vi "DSP_conditioning_Rx.bkp - Copy.vi"(4 "rx.output sample rate":fxp<+,48,1>=1.0, 5 "rx.input valid":bool, 6 "rx.frequency shift":fxp<+/-,48,0> format="%#.48g", 7 "rx.reset":bool, 8 "rx.phase":fxp<+/-,21,0>, 9 "rx.delay":fxp<+/-,16,0>, 10 "rx.impairments":T2={"inline gain I"=0.9999923706054688, "inline gain Q"=0.9999923706054688, "cross gain I"=0.0, "cross gain Q"=0.0, "pre-gain offset I"=0.0, "pre-gain offset Q"=0.0, "post-gain offset I"=0.0, "post-gain offset Q"=0.0}, 11 "IQ data":T1) -> (1 "rx.dsp reset done":bool, 2 "output valid":bool, 3 "data out":T1)   [LabVIEW 2017]
uses:
  <instrlib>/_niInstr/DSP/v1/Shared/Public/IQ Impairments.ctl
  <instrlib>/_niInstr/DSP/v1/Shared/Public/IQ Data.ctl
  <instrlib>/_niInstr/DSP/v1/FPGA/Public/Sub VIs/IQ Impairments/IQ Impairments - 1 spc.vi
  <instrlib>/_niInstr/DSP/v1/FPGA/Public/Sub VIs/Frequency Shift/Frequency Shift - 1 spc.vi
  <instrlib>/_niInstr/DSP/v1/FPGA/Public/Sub VIs/Data Conversion/IQ to U32 - 1 spc - S18.1.vi
  <instrlib>/_niInstr/DSP/v1/FPGA/niInstr DSP v1 FPGA.lvlib
  <instrlib>/_niInstr/Basic Elements/v1/FPGA/niInstr Basic Elements v1 FPGA.lvlib
  <instrlib>/_niInstr/DSP/v1/FPGA/Public/Sub VIs/Fractional Decimator/Fractional Decimator - 1 spc - 2x oc.vi
  <instrlib>/_niInstr/DSP/v1/Shared/niInstr DSP v1 Shared.lvlib
panel:
  out "U32 data":u32
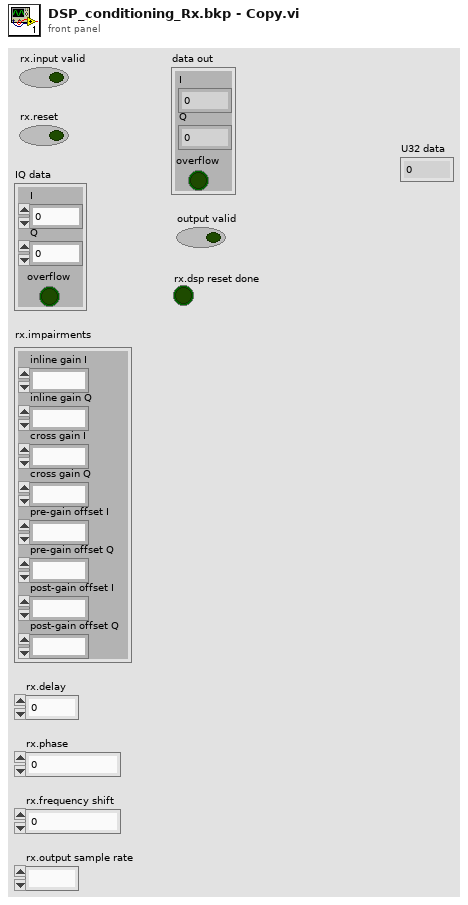
[diagram p1: front panel]
types:
  T1 = typedef "niInstr DSP v1 Shared.lvlib/IQ Data.ctl" = cluster{"I":fxp<+/-,18,1>, "Q":fxp<+/-,18,1>, "overflow":bool}
  T2 = typedef "niInstr DSP v1 Shared.lvlib/IQ Impairments.ctl" = cluster{"inline gain I":fxp<+/-,18,1>, "inline gain Q":fxp<+/-,18,1>, "cross gain I":fxp<+/-,18,1>, "cross gain Q":fxp<+/-,18,1>, "pre-gain offset I":fxp<+/-,18,1>, "pre-gain offset Q":fxp<+/-,18,1>, "post-gain offset I":fxp<+/-,18,1>, "post-gain offset Q":fxp<+/-,18,1>}
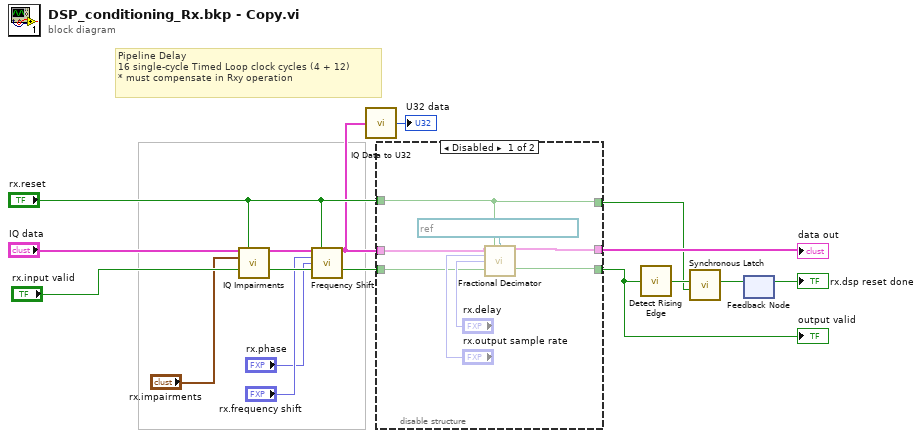
[diagram p0: block diagram]
diagram:
  # "Pipeline Delay \n16 single-cycle Timed Loop clock cycles (4 + 12)\n* must compensate in Rxy operation"
  n1 = call-poly <instrlib>:"IQ Impairments.vi"("data in"="IQ data", "reset"="rx.reset", "impairments"="rx.impairments", "input valid"="rx.input valid") -> ("data out"=w3:T1, "output valid"=w8:bool)  [unwired: 9 in, 1 out]
  n2 = call-poly <instrlib>:"Frequency Shift.vi"("data in"=w3, "reset"="rx.reset", "frequency shift"="rx.frequency shift", "phase"="rx.phase", "input valid"=w8) -> ("data out"=w2:T1, "output valid"=w4:bool)  [unwired: 8 in, 1 out]
  n3 = call-poly <instrlib>:"IQ Data to U32.vi"("IQ data"=w2) -> ("U32 data"=→"U32 data":u32)  [unwired: 13 in, 1 out]
  n4 = disable-structure shown="Disabled" {
    disable-tunnel: w2 -> [w22 w28]
    disable-tunnel: [w21 w28] -> w14
    disable-tunnel: w4 -> [w20 w27]
    disable-tunnel: "rx.reset" -> [w18 w26]
    disable-tunnel: [w19 w27] -> w10
    disable-tunnel: [w18 w26] -> w9
    frame Disabled {
      n5 = call-poly <instrlib>:"Fractional Decimator.vi"("data in"=w22, "reset"=w18, "clock x 2"=refnum<k21> "IO Module\\Data Clock x2", "output sample rate"="rx.output sample rate", "delay"="rx.delay", "input valid"=w20) -> ("data out"=w21:T1, "output valid"=w19:bool)  [unwired: 7 in, 1 out]
    }
    frame Enabled {
    }
  }
  "data out" <- w14
  "output valid" <- w10
  n6 = call <instrlib>:"Detect Rising Edge.vi"("signal"=w10) -> ("edge detected"=w12:bool)  [unwired: 14 in]
  n7 = call <instrlib>:"Synchronous Latch.vi"("clear"=w9, "set"=w12) -> ("out"=w13:bool)  [unwired: 9 in]
  n8 = feedback #1() -> (→"rx.dsp reset done":bool)  [unwired: 1 in]
  n9 = feedback-in #1(w13) -> ()
